vi "LSCI332 ErrorHandler.vi"(2 "error in (no error)":errorcluster) -> (0 "error out":errorcluster, 1 "Erreur":bool)   [LabVIEW 2019]
doc: "Ce VI vérifie si une erreur a eu lieu et si c'est le cas, il affiche un message. Si l'erreur provient du contrôleur, celle-ci est ensuite effacée."
uses:
  <vilib>/Utility/error.llb/DialogType.ctl
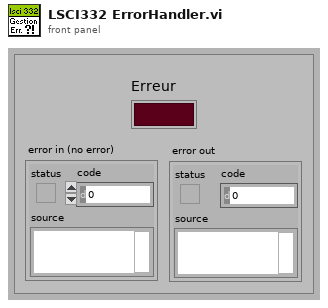
[diagram p1: front panel]
types:
  T1 = typedef "DialogType.ctl" = u16
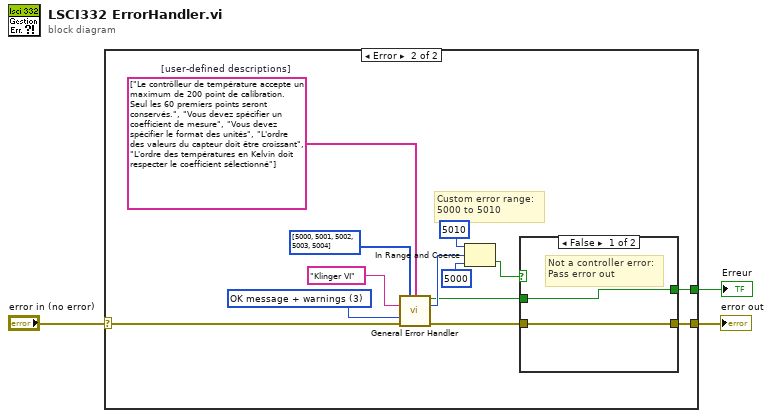
[diagram p0: block diagram]
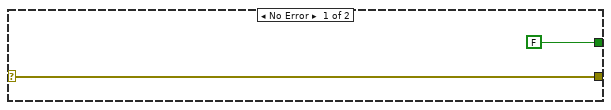
[diagram p2: hidden frame]
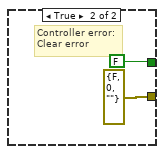
[diagram p3: hidden frame]
diagram:
  n1 = case shown="Error" "error in (no error)" {
    selector: "error in (no error)" -> [w5 w15]
    tunnel: [w5 w13] -> w3
    tunnel: [FALSE ("error?") w8] -> w2
    frame No Error {
    }
    frame Error {
      w6 = string[] ["Le contrôlleur de température accepte un maximum de 200 point de calibration. Seul les 60 premiers points seront conservés.", "Vous devez spécifier un coefficient de mesure", "Vous devez spécifier le format des unités", "L'ordre des valeurs du capteur doit être croissant", "L'ordre des températures en Kelvin doit respecter le coefficient sélectionné"]  # [user-defined descriptions]
      w18 = T1 3 items=["no dialog", "OK message", "continue or stop message", "OK message + warnings", "continue/stop + warnings"] ("type of dialog (OK msg:1)")
      # "Custom error range:\n5000 to 5010"
      n2 = call <vilib>:"General Error Handler.vi"("[user-defined codes]"=i32[] [5000, 5001, 5002, 5003, 5004], "[user-defined descriptions]"=w6, "[error source] (\" \")"="Klinger VI" ("[error source] (\" \")"), "type of dialog (OK msg:1)"=w18, "error in (no error)"=w15) -> ("error?"=w7:bool, "code out"=w12:i32, "error out"=w14:errorcluster)  [unwired: 6 in, 2 out]
      n3 = In Range and Coerce(upper limit=5010, x=w12, lower limit=5000) -> (In Range?=w9:bool)  [unwired: 1 out]
      n4 = case shown="False" w9 {
        tunnel: [w20 errorcluster {"status"=FALSE, "code"=0, "source"=""} ("error out")] -> w13
        tunnel: w14 -> [w20 _]
        tunnel: [w19 FALSE ("error?")] -> w8
        tunnel: w7 -> [w19 _]
        frame False {
          # "Not a controller error:\nPass error out"
        }
        frame True {
          # "Controller error:\nClear error"
        }
      }
    }
  }
  "Erreur" <- w2
  "error out" <- w3
